vi "多通道CAN 回读.vi"(6 "传感器选择":enum16{"CAB500", "CAB1500"}(ring), 8 "错误输入（无错误）":errorcluster, 10 "Delay Time (s)":dbl=0.2 format="%#_13g") -> (0 "错误输出":errorcluster, 1 "解析电流":dbl, 2 "报文数组":string, 3 "十次平均":dbl)   [LabVIEW 2021]
uses:
  <userlib>/PCANBasic/PCANBasic.lvlib
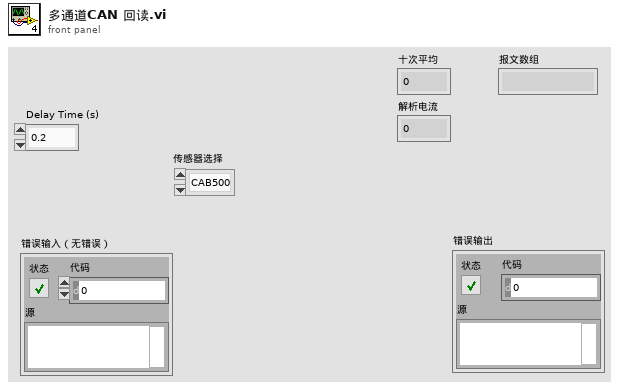
[diagram p1: front panel]
types:
  T1 = cluster{"ID":u32, "MSGTYPE":u8, "LEN":u8, "DATA[0]":u8, "DATA[1]":u8, "DATA[2]":u8, "DATA[3]":u8, "DATA[4]":u8, "DATA[5]":u8, "DATA[6]":u8, "DATA[7]":u8}
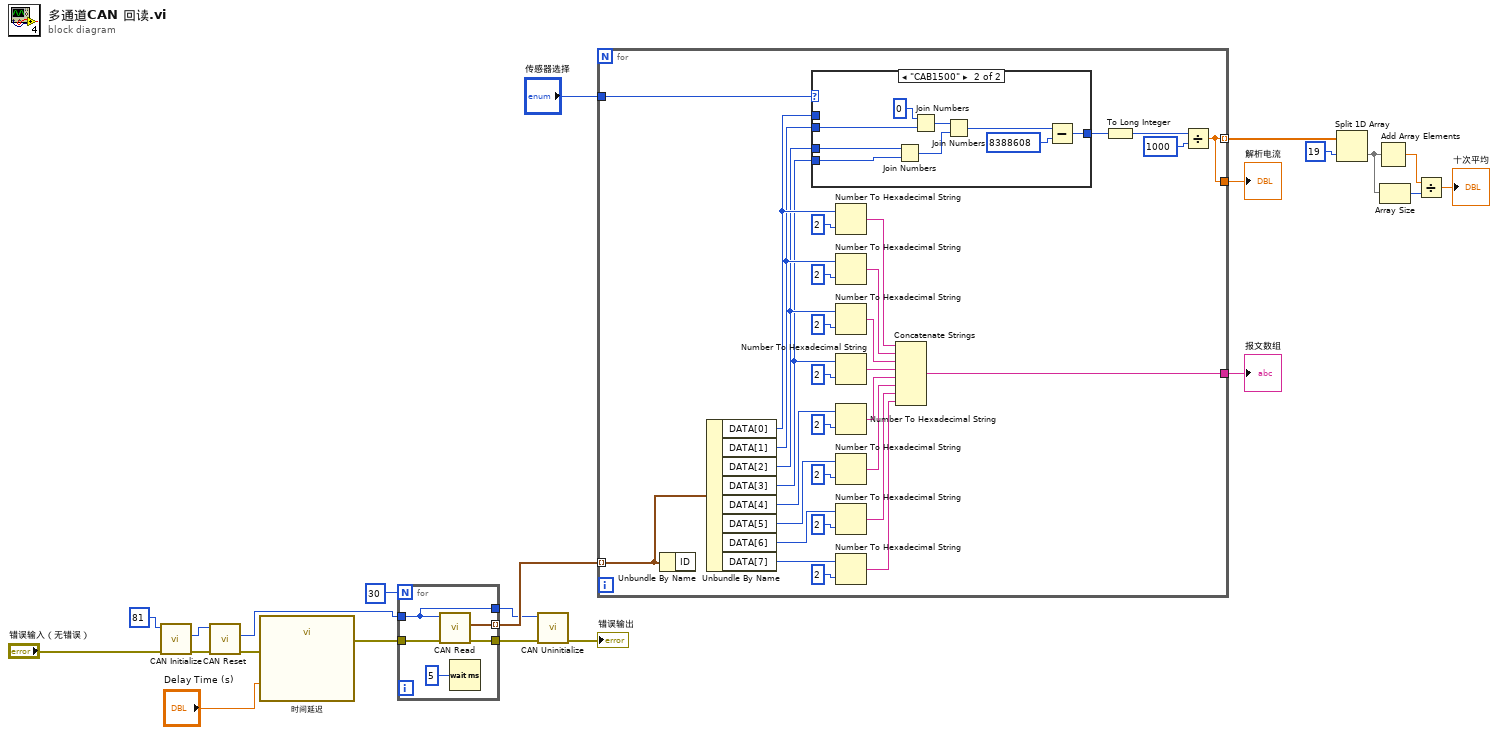
[diagram p0: block diagram]
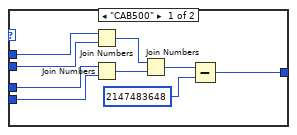
[diagram p2: hidden frame]
diagram:
  n1 = call "CAN Initialize.vi"("错误输入（无错误）"="错误输入（无错误）", "Channel"=u16 81) -> ("错误输出"=w16:errorcluster, "Channel out"=w11:u16)  [unwired: 7 in, 1 out]
  n2 = call "CAN Reset.vi"("错误输入（无错误）"=w16, "Channel in"=w11) -> ("错误输出"=w14:errorcluster, "Channel out"=w17:u16)  [unwired: 7 in, 1 out]
  n3 = call "时间延迟"("error in (no error)"=w14, "Delay Time (s)"="Delay Time (s)") -> ("error out"=w13:errorcluster)  [unwired: 9 in]
  n4 = for {
    N: 30 -> [_]
    tunnel: w17 -> [w25]
    tunnel: [w26] -> w19 mode=indexing
    tunnel: [w25] -> w18
    tunnel: w13 -> [w24]
    tunnel: [w23] -> w15
    n5 = call <userlib>:"CAN Read.vi"("error in (no error)"=w24, "Channel"=w25) -> ("error out"=w23:errorcluster, "MessageBuffer out"=w26:T1)  [unwired: 6 in, 2 out]
    n6 = Wait (ms)(milliseconds to wait=u32 5 ("等待时间（毫秒）")) -> ()  [unwired: 1 out]
  }
  n7 = call <userlib>:"CAN Uninitialize.vi"("错误输入（无错误）"=w15, "Channel"=w18) -> ("错误输出"=→"错误输出":errorcluster)  [unwired: 7 in, 2 out]
  n8 = for {
    tunnel: w19 -> [w58] mode=indexing
    tunnel: [w54] -> w4 mode=indexing
    tunnel: [w54] -> w8
    tunnel: [w29] -> w7
    tunnel: "传感器选择" -> [w28]
    n9 = Unbundle By Name(w58) -> ()  [unwired: 1 out]
    n10 = Unbundle By Name(w58) -> ("DATA[0]"=w53:u8, "DATA[1]"=w46:u8, "DATA[2]"=w45:u8, "DATA[3]"=w44:u8, "DATA[4]"=w43:u8, "DATA[5]"=w42:u8, "DATA[6]"=w39:u8, "DATA[7]"=w38:u8)
    n11 = case shown="\"CAB1500\"" w28 {
      tunnel: [w63 w74] -> w57
      tunnel: w53 -> [w62 _]
      tunnel: w46 -> [w61 w70]
      tunnel: w45 -> [w60 w69]
      tunnel: w44 -> [w59 w68]
      frame "CAB500" {
        n12 = Join Numbers(hi=w62, lo=w61) -> ((hi.lo)=w64:u16)
        n13 = Join Numbers(hi=w60, lo=w59) -> ((hi.lo)=w66:u16)
        n14 = Join Numbers(hi=w64, lo=w66) -> ((hi.lo)=w65:u32)
        n15 = Subtract(x=w65, y=u32 2147483648) -> (x-y=w63:u32)
      }
      frame "CAB1500" {
        n16 = Join Numbers(hi=w69, lo=w68) -> ((hi.lo)=w75:u16)
        n17 = Join Numbers(hi=u8 0, lo=w70) -> ((hi.lo)=w72:u16)
        n18 = Join Numbers(hi=w72, lo=w75) -> ((hi.lo)=w73:u32)
        n19 = Subtract(x=w73, y=u32 8388608) -> (x-y=w74:u32)
      }
    }
    n20 = Number To Hexadecimal String(1:i16 2 ("宽度(-)"), 2:w53) -> (0:w37:string)
    n21 = Number To Hexadecimal String(1:i16 2 ("宽度(-)"), 2:w46) -> (0:w36:string)
    n22 = Number To Hexadecimal String(1:i16 2 ("宽度(-)"), 2:w45) -> (0:w35:string)
    n23 = Number To Hexadecimal String(1:i16 2 ("宽度(-)"), 2:w44) -> (0:w34:string)
    n24 = Number To Hexadecimal String(1:i16 2 ("宽度(-)"), 2:w43) -> (0:w33:string)
    n25 = Number To Hexadecimal String(1:i16 2 ("宽度(-)"), 2:w42) -> (0:w32:string)
    n26 = Number To Hexadecimal String(1:i16 2 ("宽度(-)"), 2:w39) -> (0:w31:string)
    n27 = Number To Hexadecimal String(1:i16 2 ("宽度(-)"), 2:w38) -> (0:w30:string)
    n28 = Concatenate Strings(w37, w36, w35, w34, w33, w32, w31, w30) -> (w29:string)
    n29 = To Long Integer(number=w57) -> (32bit integer=w56:i32)
    n30 = Divide(x=w56, y=1000) -> (x/y=w54:dbl)
  }
  "解析电流" <- w8
  "报文数组" <- w7
  n31 = Split 1D Array(array=w4, index=19 ("索引")) -> (second subarray=w2:dbl[])  [unwired: 1 out]
  n32 = Add Array Elements(numeric array=w2) -> (sum=w1:dbl)
  n33 = Array Size(array=w2) -> (size(s)=w10:i32)
  n34 = Divide(x=w1, y=w10) -> (x/y=→"十次平均":dbl)
